vi "Main.vi"() -> ()   [LabVIEW 2020, in "Nested.lvlib"]
uses:
  Nested.lvlib
  OOPanel/Manager/Manager.lvclass
  ArrayHostPanel/ArrayHostPanel.lvclass
panel:
  out "error out":errorcluster
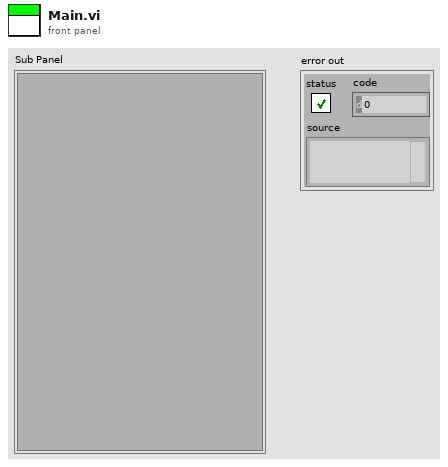
[diagram p1: front panel]
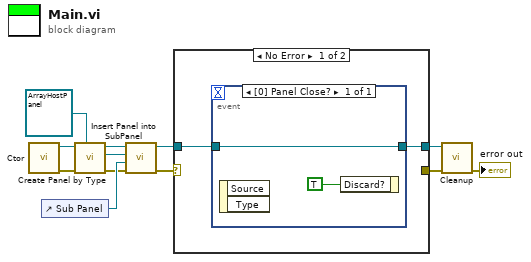
[diagram p0: block diagram]
diagram:
  n1 = call "Ctor.vi"() -> ("error out"=w5:errorcluster, "Manager out"=w6:refnum<class "Manager.lvclass">)  [unwired: 10 in]
  n2 = control-ref of="Sub Panel"() -> (w12:refnum<vi>)
  n3 = call "Create Panel by Type.vi"("Panel Type"=refnum<class "ArrayHostPanel.lvclass"> refnum ("Nested.lvlib:ArrayHostPanel.lvclass"), "error in (no error)"=w5, "Manager in"=w6) -> ("error out"=w3:errorcluster, "Panel"=w1:refnum<class "ArrayHostPanel.lvclass">, "Manager out"=w4:refnum<class "Manager.lvclass">)  [unwired: 6 in]
  n4 = call "Insert Panel into SubPanel.vi"("error in (no error)"=w3, "SubPanel"=w12, "Panel In"=w1, "Manager in"=w4) -> ("error out"=w9:errorcluster, "Manager out"=w11:refnum<class "Manager.lvclass">)  [unwired: 5 in, 1 out]
  n5 = case shown="No Error" w9 {
    selector: w9 -> [_ w18]
    tunnel: w11 -> [w14 w17]
    tunnel: [w13 w17] -> w10
    tunnel: [_ w18] -> w8
    frame No Error {
      n6 = event shown="[0] Panel Close?" {
        selector: _ -> [_]
        dyn-events: _ -> [_]
        timeout: _ -> [_]
        tunnel: w14 -> [w15]
        tunnel: [w15] -> w13
        event Panel Close? {
          n7 = event-data() -> ()  [unwired: 1 in, 2 out]
          n8 = event-data("Discard?"=TRUE) -> ()  [unwired: 1 in, 1 out]
        }
      }
    }
    frame Error {
    }
  }
  n9 = call "Cleanup.vi"("error in (no error)"=w8, "Manager in"=w10) -> ("error out"=→"error out":errorcluster)  [unwired: 7 in, 2 out]
